vi "lab1_example_sine_signal_generator_v2.vi"() -> ()   [LabVIEW 2014]
uses:
  <vilib>/addons/Modulation/Analog/controls/Complex Data Waveform.ctl
  <vilib>/Analysis/1siggen.llb/Ramp Pattern by Samples.vi
  sub_var_stop.vi
  <vilib>/measure/maspectr.llb/FFT Power Spectrum and PSD for 1 Chan (CDB).vi
  <vilib>/addons/Modulation/niAMT.lvlib
  <vilib>/Analysis/NI_AALBase.lvlib
  <vilib>/measure/NI_MAPro.lvlib
panel:
  out "Waveform Graph":cluster{"f0":dbl, "df":dbl, "magnitude":dbl[]}(graph)
  in  "sampling rate":dbl format="%#_13g"
  in  "frequency":dbl format="%#_13g"
  in  "duration":dbl format="%#_13g"
  in  "stop":bool
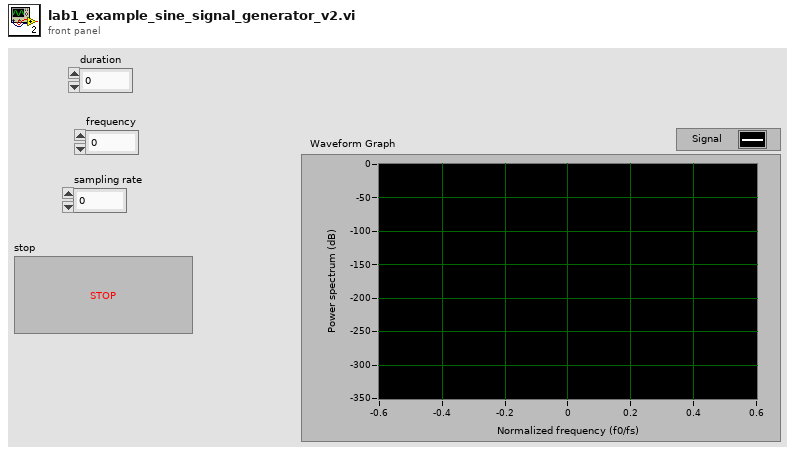
[diagram p1: front panel]
types:
  T1 = typedef "niAMT.lvlib/Complex Data Waveform.ctl" = cluster{"t0":dbl, "dt":dbl, "Y":cdb[]}
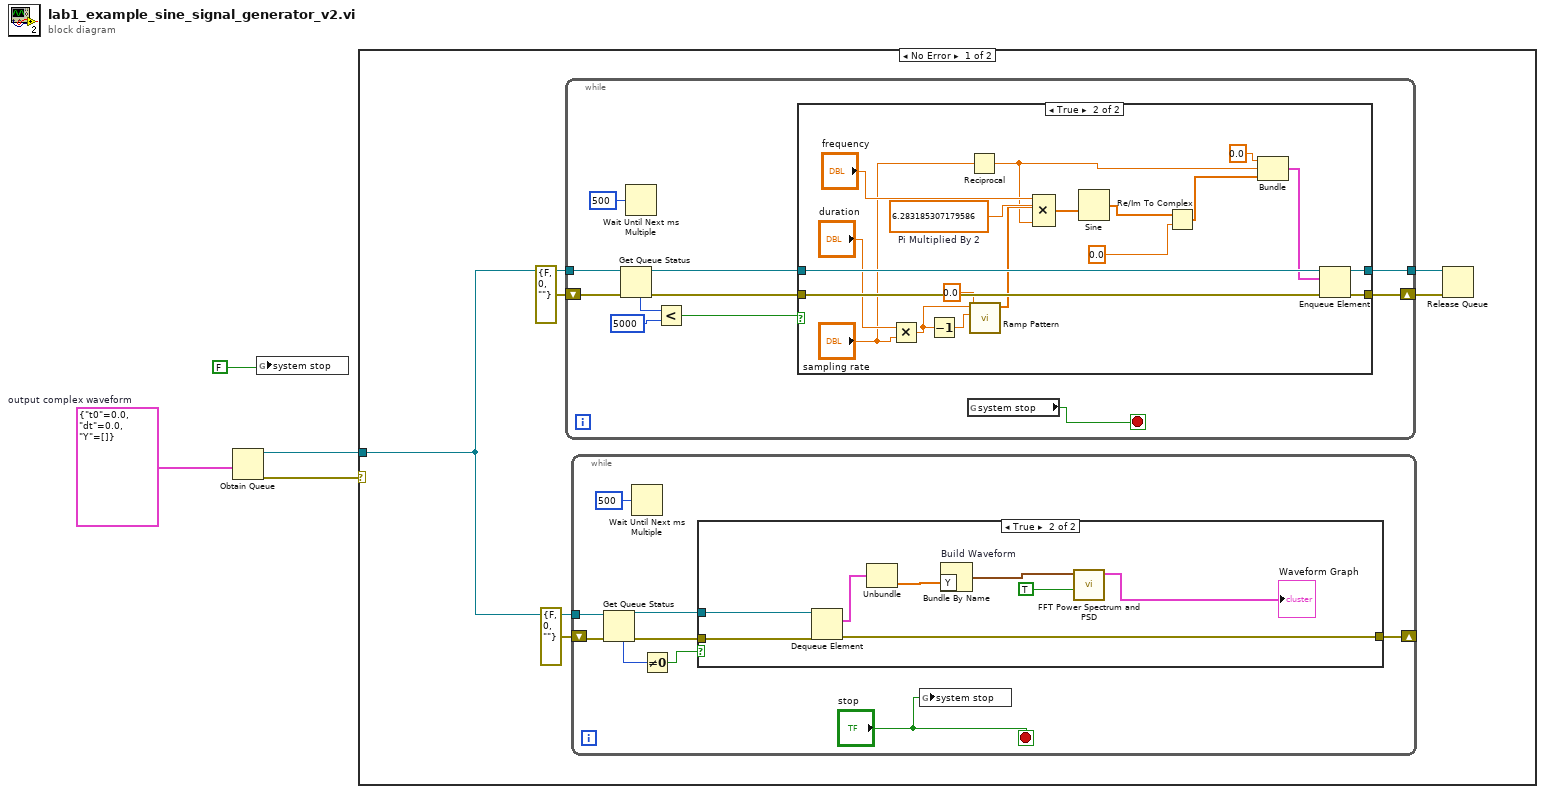
[diagram p0: block diagram]
diagram:
  w2 = T1 {"t0"=0.0, "dt"=0.0, "Y"=[]}  # output complex waveform
  n1 = Obtain Queue(element data type=w2) -> (queue out=w1:refnum<queue>, error out=w3:errorcluster)  [unwired: 4 in, 1 out]
  n2 = global write "sub_var_stop.vi" "system stop"(FALSE) -> ()
  n3 = case shown="No Error" w3 {
    tunnel: w1 -> [w9 _]
    frame No Error {
      n4 = while {
        tunnel: w9 -> [w37]
        shift-right: [w31] -> w7
        shift-left: errorcluster {"status"=FALSE, "code"=0, "source"=""} ("error out") -> [w36]
        tunnel: [w30] -> w6
        stop <- w38 stop-if-true
        n5 = Get Queue Status(queue=w37, error in (no error)=w36) -> (queue out=w32:refnum<queue>, error out=w33:errorcluster, # elements in queue=w35:i32)  [unwired: 1 in, 5 out]
        n6 = Wait Until Next ms Multiple(millisecond multiple=u32 500) -> ()  [unwired: 1 out]
        n7 = Less?(x=w35, y=5000) -> (x < y?=w28:bool)
        n8 = case shown="True" w28 {
          tunnel: w33 -> [w40 w59]
          tunnel: w32 -> [w39 w58]
          tunnel: [w40 w57] -> w31
          tunnel: [w39 w56] -> w30
          frame False {
          }
          frame True {
            w51 = 6.283185307179586  # Pi Multiplied By 2
            n9 = Multiply(x="duration", y="sampling rate") -> (x*y=w54:dbl)
            n10 = Decrement(x=w54) -> (x-1=w53:dbl)
            n11 = Reciprocal(x="sampling rate") -> (1/x=w41:dbl)
            n12 = call-poly <vilib>:"Ramp Pattern.vi"("start"=0.0, "end"=w53, "samples"=w54) -> ("Ramp Pattern"=w50:dbl[])  [unwired: 7 in, 1 out]
            n13 = Compound Arithmetic op=MULTIPLY("frequency", w50, w51, w41) -> (w48:dbl[])
            n14 = Sine(x=w48) -> (sin(x)=w47:dbl[])
            n15 = Re/Im To Complex(1:0.0, 2:w47) -> (0:w45:cdb[])
            n16 = Bundle "Bundle"(0.0, w41, w45) -> (w42:cluster{dbl, dbl, cdb[]})  [unwired: 1 in]
            n17 = Enqueue Element(queue=w58, element=w42, error in (no error)=w59) -> (queue out=w56:refnum<queue>, error out=w57:errorcluster)  [unwired: 1 in, 1 out]
          }
        }
        n18 = global read "sub_var_stop.vi" "system stop"() -> (w38:bool)
      }
      n19 = while {
        tunnel: w9 -> [w17]
        shift-right: [w11] -> _
        shift-left: errorcluster {"status"=FALSE, "code"=0, "source"=""} ("error out") -> [w16]
        stop <- "stop" stop-if-true
        n20 = Get Queue Status(queue=w17, error in (no error)=w16) -> (queue out=w12:refnum<queue>, error out=w13:errorcluster, # elements in queue=w15:i32)  [unwired: 1 in, 5 out]
        n21 = Wait Until Next ms Multiple(millisecond multiple=u32 500) -> ()  [unwired: 1 out]
        n22 = Not Equal To 0?(x=w15) -> (x != 0?=w14:bool)
        n23 = case shown="True" w14 {
          tunnel: w13 -> [w19 w27]
          tunnel: w12 -> [_ w26]
          tunnel: [w19 w25] -> w11
          frame False {
          }
          frame True {
            n24 = Dequeue Element(queue=w26, error in (no error)=w27) -> (element=w24:T1, error out=w25:errorcluster)  [unwired: 1 in, 2 out]
            n25 = Unbundle "Unbundle"(w24) -> ("Y"=w23:cdb[])  [unwired: 2 out]
            n26 = Bundle By Name "Build Waveform"("Y"=w23) -> (w22:waveform(cdb))  [unwired: 1 in]
            n27 = call-poly <vilib>:"FFT Power Spectrum and PSD.vi"("dB On (F)"=TRUE, "time signal"=w22) -> ("Power Spectrum / PSD"=→"Waveform Graph":cluster{"f0":dbl, "df":dbl, "magnitude":dbl[]})  [unwired: 6 in, 3 out]
          }
        }
        n28 = global write "sub_var_stop.vi" "system stop"("stop") -> ()
      }
      n29 = Release Queue(queue=w6, error in (no error)=w7) -> ()  [unwired: 1 in, 3 out]
    }
    frame Error {
    }
  }
